vi "Riccati_DARE_N.vi"(6 "N":T1, 8 "R":T1, 9 "Q":T1, 10 "B":T1, 11 "A":T1) -> (0 "error out":errorcluster, 1 "Error":bool, 2 "Iterations":i32, 3 "Answer":T1)   [LabVIEW 2019, in "Trajectory_Library.lvlib"]
doc: "Solves the discrete alegebraic Riccati equation.\n \nInput:\n - A -- System matrix.\n - B -- nput matrix.\n - Q -- State cost matrix.\n - R -- Input cost matrix.\n - N -- State-input cross-term cost matrix.\n\nOutputs:\n Answer -- Solution of DARE.\n iterations -- Number of iterations\n error -- If TRUE, an error occured\n\nSee https://en.wikipedia.org/wiki/Linear%E2%80%93quadratic_regulator#Infinite-horizon,_discrete-time_LQR for the change of variables used here."
uses:
  Trajectory_Library.lvlib
  <vilib>/Analysis/Matrix/Datatypes/RealMatrix.ctl
  <vilib>/Analysis/7linalg.llb/Real Transpose Matrix.vi
  <vilib>/Analysis/baseanly.llb/Real A x B.vi
  <vilib>/Analysis/7linalg.llb/Solve Linear Equations (multiple right hand).vi
  <vilib>/Analysis/Matrix/Numeric/Subtract/Subtract - RM,RM.vi
  <vilib>/Analysis/NI_AALPro.lvlib
  <vilib>/Analysis/NI_AALBase.lvlib
  <vilib>/Analysis/Matrix/NI_Matrix.lvlib
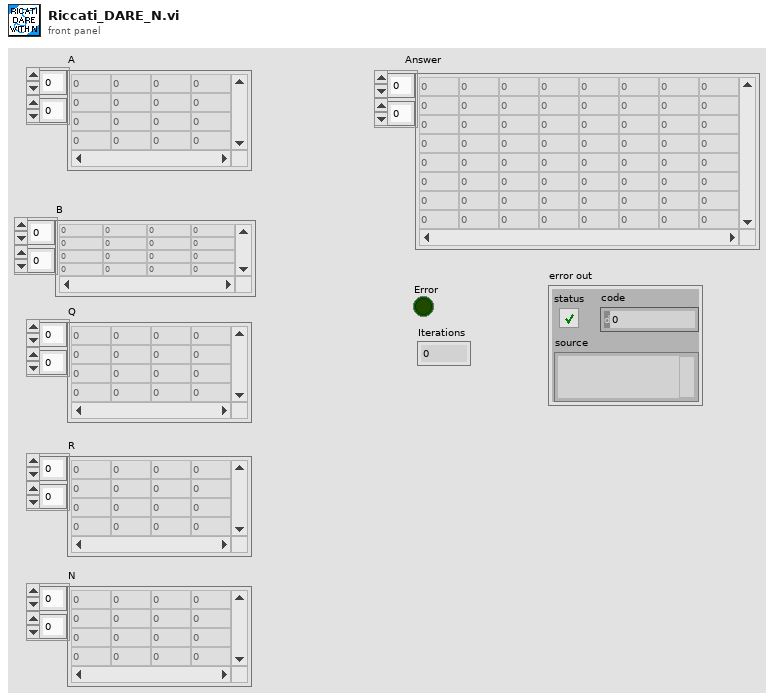
[diagram p1: front panel]
types:
  T1 = typedef "NI_Matrix.lvlib/RealMatrix.ctl" = dbl[][]
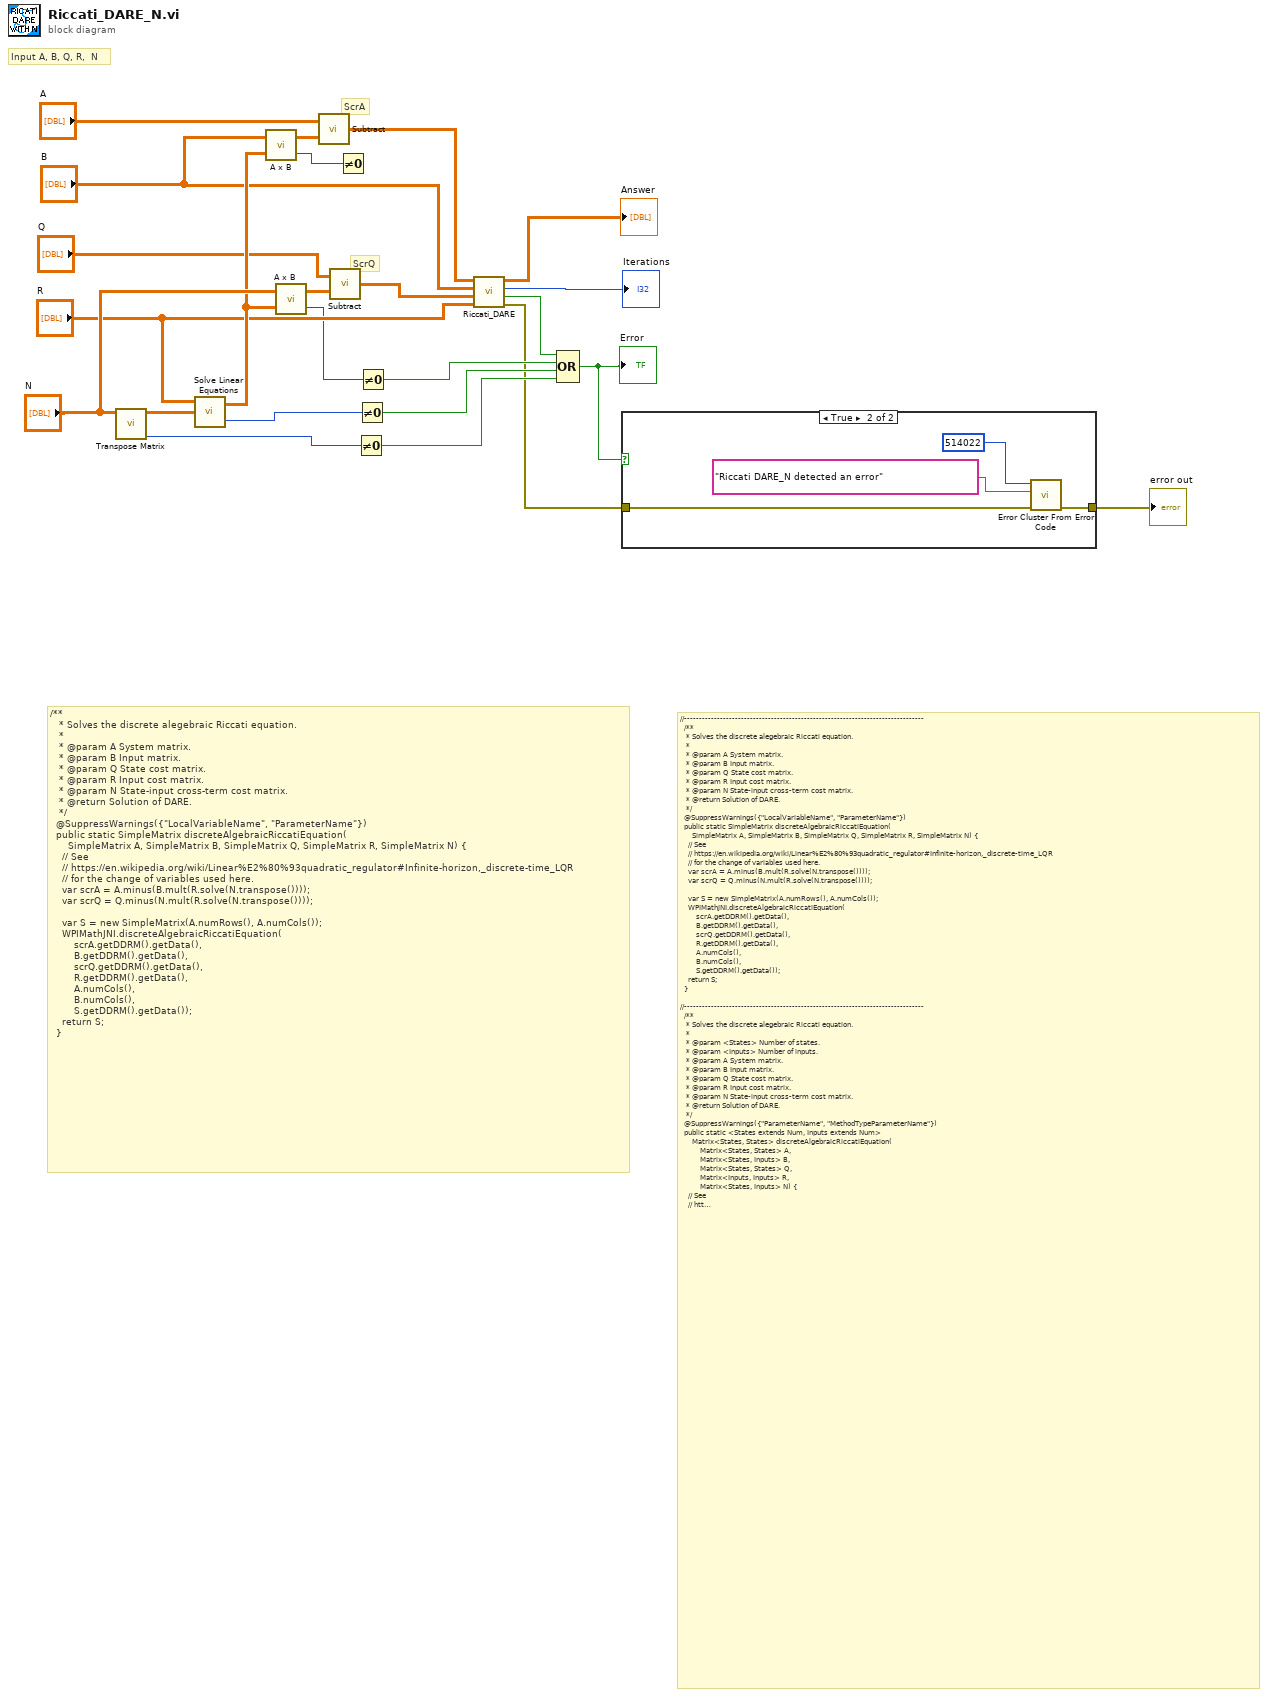
[diagram p0: block diagram]
diagram:
  # "//--------------------------------------------------------------------------------\n  /**\n   * Solves the discrete alegebraic Riccati equation.\n   *\n   * @param A System matrix.\n   * @param B Input matrix.\n   * @param Q State cost matrix.\n   * @param R Input cost matrix.\n   * @param N State-input cross-term cost matrix.\n   * @return Solution of DARE.\n   */\n  @SuppressWarnings({\"LocalVariableName\", \"ParameterName\"})\n  public static SimpleMatrix discreteAlgebraicRiccatiEquation(\n      SimpleMatrix A, SimpleMatrix B, SimpleMatrix Q, SimpleMatrix R, SimpleMatrix N) {\n    // See\n    // https://en.wikipedia.org/wiki/Linear%E2%80%93quadratic_regulator#Infinite-horizon,_discrete-time_LQR\n    // for the change of variables used here.\n    var scrA = A.minus(B.mult(R.solve(N.transpose())));\n    var scrQ = Q.minus(N.mult(R.solve(N.transpose())));\n\n    var S = new SimpleMatrix(A.numRows(), A.numCols());\n    WPIMathJNI.discreteAlgebraicRiccatiEquation(\n        scrA.getDDRM().getData(),\n        B.getDDRM().getData(),\n        scrQ.getDDRM().getData(),\n        R.getDDRM().getData(),\n        A.numCols(),\n        B.numCols(),\n        S.getDDRM().getData());\n    return S;\n  }\n\n//--------------------------------------------------------------------------------\n  /**\n   * Solves the discrete alegebraic Riccati equation.\n   *\n   * @param <States> Number of states.\n   * @param <Inputs> Number of inputs.\n   * @param A System matrix.\n   * @param B Input matrix.\n   * @param Q State cost matrix.\n   * @param R Input cost matrix.\n   * @param N State-input cross-term cost matrix.\n   * @return Solution of DARE.\n   */\n  @SuppressWarnings({\"ParameterName\", \"MethodTypeParameterName\"})\n  public static <States extends Num, Inputs extends Num>\n      Matrix<States, States> discreteAlgebraicRiccatiEquation(\n          Matrix<States, States> A,\n          Matrix<States, Inputs> B,\n          Matrix<States, States> Q,\n          Matrix<Inputs, Inputs> R,\n          Matrix<States, Inputs> N) {\n    // See\n    // https://en.wikipedia.org/wiki/Linear%E2%80%93quadratic_regulator#Infinite-horizon,_discrete-time_LQR\n    // for the change of variables used here.\n    var scrA = A.minus(B.times(R.solve(N.transpose())));\n    var scrQ = Q.minus(N.times(R.solve(N.transpose())));\n\n    return new Matrix<>(\n        discreteAlgebraicRiccatiEquation(\n            scrA.getStorage(), B.getStorage(), scrQ.getStorage(), R.getStorage()));\n  }\n}"
  # "ScrQ"
  # "ScrA"
  # "/**\n   * Solves the discrete alegebraic Riccati equation.\n   *\n   * @param A System matrix.\n   * @param B Input matrix.\n   * @param Q State cost matrix.\n   * @param R Input cost matrix.\n   * @param N State-input cross-term cost matrix.\n   * @return Solution of DARE.\n   */\n  @SuppressWarnings({\"LocalVariableName\", \"ParameterName\"})\n  public static SimpleMatrix discreteAlgebraicRiccatiEquation(\n      SimpleMatrix A, SimpleMatrix B, SimpleMatrix Q, SimpleMatrix R, SimpleMatrix N) {\n    // See\n    // https://en.wikipedia.org/wiki/Linear%E2%80%93quadratic_regulator#Infinite-horizon,_discrete-time_LQR\n    // for the change of variables used here.\n    var scrA = A.minus(B.mult(R.solve(N.transpose())));\n    var scrQ = Q.minus(N.mult(R.solve(N.transpose())));\n\n    var S = new SimpleMatrix(A.numRows(), A.numCols());\n    WPIMathJNI.discreteAlgebraicRiccatiEquation(\n        scrA.getDDRM().getData(),\n        B.getDDRM().getData(),\n        scrQ.getDDRM().getData(),\n        R.getDDRM().getData(),\n        A.numCols(),\n        B.numCols(),\n        S.getDDRM().getData());\n    return S;\n  }"
  # "Input A, B, Q, R,  N"
  n1 = call-poly <vilib>:"Transpose Matrix.vi"("Input Matrix"="N") -> ("error"=w10:i32, "Matrix Transpose"=w24:T1)  [unwired: 9 in]
  n2 = call-poly <vilib>:"Solve Linear Equations.vi"("Known Matrix"=w24, "Input Matrix"="R") -> ("error"=w11:i32, "Solution Matrix"=w20:T1)  [unwired: 1 in]
  n3 = call-poly <vilib>:"A x B.vi"("B"=w20, "A"="B") -> ("error"=w13:i32, "A x B"=w23:T1)
  n4 = call-poly <vilib>:"A x B.vi"("B"=w20, "A"="N") -> ("error"=w12:i32, "A x B"=w19:T1)
  n5 = call-poly <vilib>:"Subtract.vi"("Real Matrix B"=w23, "Real Matrix A"="A") -> ("A - B"=w17:T1)
  n6 = call-poly <vilib>:"Subtract.vi"("Real Matrix B"=w19, "Real Matrix A"="Q") -> ("A - B"=w15:T1)
  n7 = Not Equal To 0?(x=w13) -> ()  [unwired: 1 out]
  n8 = Not Equal To 0?(x=w10) -> (x != 0?=w6:bool)
  n9 = Not Equal To 0?(x=w11) -> (x != 0?=w7:bool)
  n10 = Not Equal To 0?(x=w12) -> (x != 0?=w8:bool)
  n11 = call "Riccati_DARE.vi"("R"="R", "Q"=w15, "B"="B", "A"=w17) -> ("error out"=w1:errorcluster, "Error"=w9:bool, "Iterations"=→"Iterations":i32, "Answer"=→"Answer":T1)  [unwired: 4 in]
  n12 = Compound Arithmetic op=OR(w9, w8, w7, w6) -> (w2:bool)
  "Error" <- w2
  n13 = case shown="True" w2 {
    tunnel: w1 -> [w25 w26]
    tunnel: [w25 w28] -> w3
    frame False {
    }
    frame True {
      n14 = call <vilib>:"Error Cluster From Error Code.vi"("error in (no error)"=w26, "error message (\"\")"="Riccati DARE_N detected an error" ("error message (\"\")"), "error code (0)"=514022) -> ("error out"=w28:errorcluster)  [unwired: 6 in]
    }
  }
  "error out" <- w3
